vi "cRIO Test Cell.vi"() -> ()   [LabVIEW 2021]
uses:
  <vilib>/DAQmx/read.llb/DAQmx Read (Analog 1D Wfm NChan NSamp).vi
  <vilib>/DAQmx/create/channels.llb/DAQmx Create Channel (AI-Temperature-Thermocouple).vi
  <vilib>/DAQmx/configure/timing.llb/DAQmx Timing (Sample Clock).vi
  <vilib>/DAQmx/miscellaneous.llb/DAQmx Fill In Error Info.vi
  logger/Logger.lvclass
panel:
  in  "Test Duration (Seconds)":i32=3600
  in  "Stop Test":bool
  out "file path out":path
  in  "Temperature Channels":tag="Mod1/ai0:3"
  in  "File Send Interval (Seconds)":dbl=600.0 format="%#_13g"
  in  "Send File":bool
  out "Buffer":i32
  out "Pressure":waveform(dbl)[](graph)
  out "Temperature":waveform(dbl)[](graph)
  out "Logger Iterations":i32
  out "Testing":bool
  in  "Start Test":bool
  out "error IO":errorcluster
  out "Files Sent":i32
  in  "stop":bool
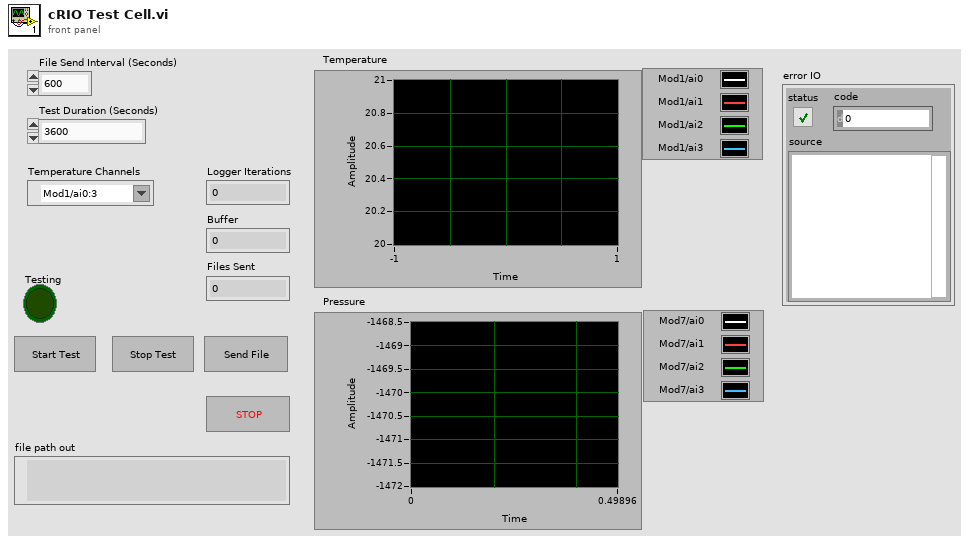
[diagram p1: front panel]
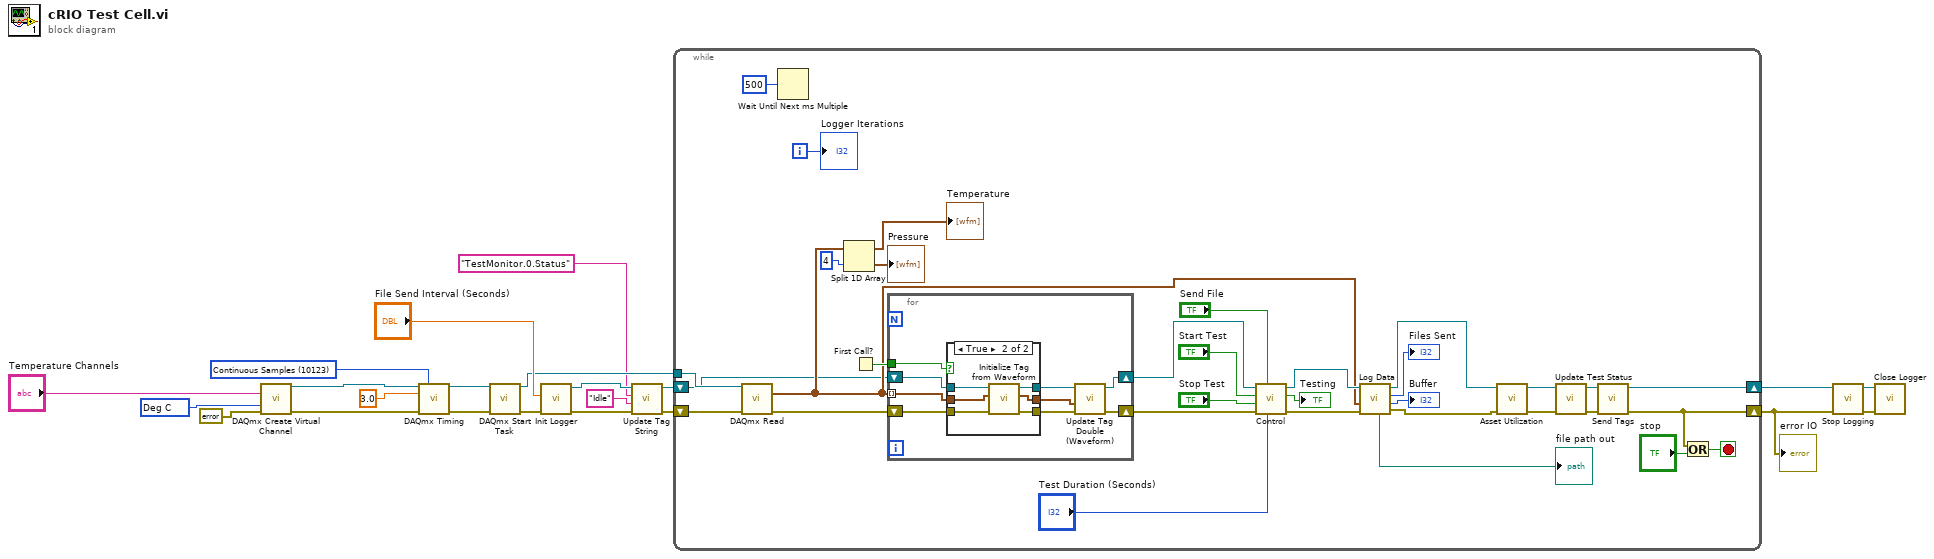
[diagram p0: block diagram]
diagram:
  w17 = 10123 items=["Finite Samples"=10178, "Continuous Samples"=10123, "Hardware Timed Single Point"=12522] ("sample mode")
  w20 = 10143 items=["Deg C"=10143, "Deg F"=10144, "Kelvins"=10325, "Deg R"=10145, "From Custom Scale"=10065] ("units")
  n1 = call-poly <vilib>:"DAQmx Create Virtual Channel.vi"("physical channels"="Temperature Channels", "units"=w20, "error in"=errorcluster {"status"=FALSE, "code"=0, "source"=""} ("error in (no error)")) -> ("task out"=w6:refnum<k21>, "error out"=w5:errorcluster)  [unwired: 11 in]
  n2 = call-poly <vilib>:"DAQmx Timing.vi"("task/channels in"=w6, "sample mode"=w17, "rate"=3.0, "error in"=w5) -> ("task out"=w19:refnum<k21>, "error out"=w18:errorcluster)  [unwired: 10 in]
  n3 = call <vilib>:"DAQmx Start Task.vi"("task/channels in"=w19, "error in"=w18) -> ("task out"=w15:refnum<k21>, "error out"=w14:errorcluster)  [unwired: 12 in]
  n4 = call "Init Logger.vi"("error in (no error)"=w14, "File Send Interval (Seconds)"="File Send Interval (Seconds)") -> ("error out"=w12:errorcluster, "Logger out.lvclass"=w11:refnum<class "Logger.lvclass">)  [unwired: 8 in]
  n5 = call "Update Tag String.vi"("error in (no error)"=w12, "string"="Idle", "Tag Path"="TestMonitor.0.Status", "Logger in.lvclass"=w11) -> ("error out"=w7:errorcluster, "Logger out.lvclass"=w8:refnum<class "Logger.lvclass">)  [unwired: 6 in]
  n6 = while {
    shift-right: [w52] -> w1
    shift-left: w7 -> [w29]
    shift-right: [w53] -> w2
    shift-left: w8 -> [w30]
    tunnel: w15 -> [w36]
    i -> [w49]
    stop <- w54 stop-if-true
    n7 = call-poly <vilib>:"DAQmx Read.vi"("task/channels in"=w36, "error in"=w29) -> ("data"=w37:waveform(dbl)[], "error out"=w35:errorcluster)  [unwired: 11 in, 1 out]
    n8 = Wait Until Next ms Multiple(millisecond multiple=u32 500) -> ()  [unwired: 1 out]
    n9 = Split 1D Array(array=w37, index=4) -> (first subarray=→"Temperature":waveform(dbl)[], second subarray=→"Pressure":waveform(dbl)[])
    n10 = First Call?() -> (First Call?: T/F=w50:bool)
    n11 = for {
      shift-right: [w63] -> w43
      shift-left: w35 -> [w60]
      shift-right: [w64] -> w44
      shift-left: w30 -> [w62]
      tunnel: w37 -> [w61] mode=indexing
      tunnel: w50 -> [w56]
      n12 = case shown="True" w56 {
        tunnel: w62 -> [w67 w73]
        tunnel: w61 -> [w66 w72]
        tunnel: w60 -> [w65 w71]
        tunnel: [w67 w70] -> w59
        tunnel: [w65 w69] -> w58
        tunnel: [w66 w68] -> w57
        frame False {
        }
        frame True {
          n13 = call "Initialize Tag from Waveform.vi"("error in (no error)"=w71, "Waveform in"=w72, "Logger in.lvclass"=w73) -> ("error out"=w69:errorcluster, "Waveform out"=w68:waveform(dbl), "Logger out.lvclass"=w70:refnum<class "Logger.lvclass">)  [unwired: 6 in]
        }
      }
      n14 = call "Update Tag Double (Waveform).vi"("error in (no error)"=w58, "Waveform"=w57, "Logger in.lvclass"=w59) -> ("error out"=w63:errorcluster, "Logger out.lvclass"=w64:refnum<class "Logger.lvclass">)  [unwired: 7 in]
    }
    n15 = call "Control.vi"("Test Duration (Seconds)"="Test Duration (Seconds)", "Send File"="Send File", "error in (no error)"=w43, "Stop Test"="Stop Test", "Start Test"="Start Test", "Logger in.lvclass"=w44) -> ("error out"=w41:errorcluster, "Testing"=→"Testing":bool, "Logger out.lvclass"=w42:refnum<class "Logger.lvclass">)  [unwired: 3 in]
    n16 = call "Log Data.vi"("error in (no error)"=w41, "Data"=w37, "Logger in.lvclass"=w42) -> ("error out"=w24:errorcluster, "Buffer"=→"Buffer":i32, "Files Sent"=→"Files Sent":i32, "Logger out.lvclass"=w23:refnum<class "Logger.lvclass">, "file path out"=→"file path out":path)  [unwired: 4 in]
    n17 = call "Asset Utilization.vi"("error in (no error)"=w24, "Logger in.lvclass"=w23) -> ("error out"=w25:errorcluster, "Logger out.lvclass"=w26:refnum<class "Logger.lvclass">)  [unwired: 8 in]
    n18 = call "Update Test Status.vi"("error in (no error)"=w25, "Logger in.lvclass"=w26) -> ("error out"=w27:errorcluster, "Logger out.lvclass"=w28:refnum<class "Logger.lvclass">)  [unwired: 8 in]
    n19 = call "Send Tags.vi"("error in (no error)"=w27, "Logger in.lvclass"=w28) -> ("error out"=w52:errorcluster, "Logger out.lvclass"=w53:refnum<class "Logger.lvclass">)  [unwired: 8 in]
    n20 = Or(x=w52, y="stop") -> (x .or. y?=w54:bool)
    "Logger Iterations" <- w49
  }
  "error IO" <- w1
  n21 = call "Stop Logging.vi"("error in (no error)"=w1, "Logger in.lvclass"=w2) -> ("error out"=w3:errorcluster, "Logger out.lvclass"=w4:refnum<class "Logger.lvclass">)  [unwired: 8 in]
  n22 = call "Close Logger.vi"("error in (no error)"=w3, "Logger in.lvclass"=w4) -> ()  [unwired: 9 in, 1 out]
